vi "write IKGMS file.vi"(9 "Corrected Array in":dbl[][](array[numeric]), 10 "Generate Array Calc IK":bool, 11 "Path in":refnum<vi>) -> (3 "appended path":path)   [LabVIEW 2016]
uses:
  <userlib>/_OpenG.lib/file/file.llb/Strip Path - Traditional__ogtk.vi
  <userlib>/_OpenG.lib/file/file.llb/Build Path - Traditional__ogtk.vi
  <vilib>/Utility/file.llb/Write Delimited Spreadsheet (DBL).vi
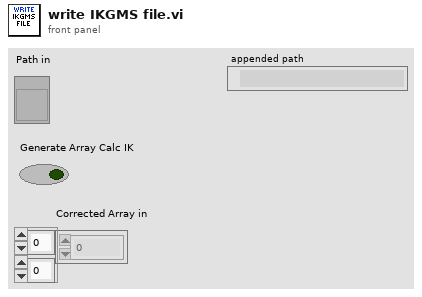
[diagram p1: front panel]
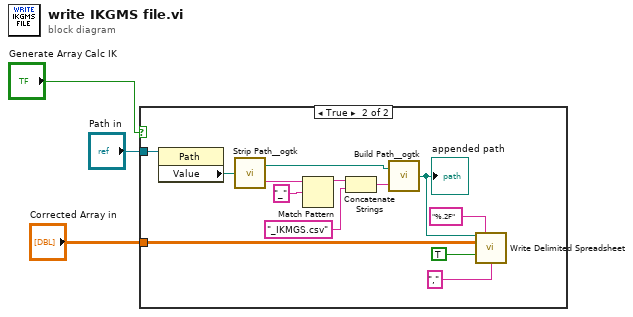
[diagram p0: block diagram]
diagram:
  n1 = case shown="True" "Generate Array Calc IK" {
    tunnel: "Corrected Array in" -> [_ w16]
    tunnel: "Path in" -> [_ w4]
    frame False {
    }
    frame True {
      n2 = property class="Path"(reference=w4) -> ("Value"=w6:path)  [unwired: 1 in, 2 out]
      n3 = call-poly <userlib>:"Strip Path__ogtk.vi"("path"=w6) -> ("stripped path"=w13:path, "name"=w11:string)
      n4 = Match Pattern(string=w11, regular expression="_") -> (before substring=w9:string)  [unwired: 1 in, 3 out]
      n5 = Concatenate Strings(w9, "_IKMGS.csv") -> (w8:string)
      n6 = call-poly <userlib>:"Build Path__ogtk.vi"("name or relative path"=w8, "base path"=w13) -> ("appended path"=w12:path)
      "appended path" <- w12
      n7 = call-poly <vilib>:"Write Delimited Spreadsheet.vi"("file path (dialog if empty)"=w12, "format (%.3f)"="%.2F", "2D data"=w16, "append to file? (new file:F)"=TRUE, "delimiter (\\t)"="," ("delimiter (\\t)")) -> ()  [unwired: 9 in, 2 out]
    }
  }
